vi "Test Find Class from Library.vi"(8 "error in (no error)":errorcluster, 11 "Test Finder Test in":refnum<class "Test Finder Test.lvclass">) -> (0 "error out":errorcluster, 3 "Test Finder Test out":refnum<class "Test Finder Test.lvclass">)   [LabVIEW 2020, in "LUnit Tests.lvlib" / "Test Finder Test.lvclass"]
uses:
  Test Finder Test.lvclass
  C:/Program Files (x86)/National Instruments/LabVIEW 2020/vi.lib/Astemes/LUnit/Test Case.lvclass
  source/Framework/Helper Classes/Test Finder/Test Finder.lvclass
  Test Dummys/Dummy Library/Test Test Case.lvclass
  <vilib>/Astemes/LUnit/Test Case.lvclass/Test Case.ctl
  <vilib>/Astemes/LUnit/LUnit Assertion Result.lvclass/LUnit Assertion Result.ctl
  <vilib>/Astemes/LUnit/LUnit Test Case Result.lvclass/LUnit Test Case Result.ctl
  <vilib>/Astemes/LUnit/LUnit Method Result.lvclass/LUnit Method Result.ctl
  <vilib>/Astemes/LUnit/Palette/Fail.vi
  <vilib>/Astemes/LUnit/Palette/Pass.vi
  <vilib>/Astemes/LUnit/Set Assertion Type.vi
  <vilib>/Astemes/LUnit/Add test result.vi
  <vilib>/Astemes/LUnit/LUnit Write Passed.vi
  <vilib>/Astemes/LUnit/LUnit Write Message.vi
  <vilib>/Astemes/LUnit/LUnit Write Description.vi
  <vilib>/Astemes/LUnit/LUnit Write Assertion Type.vi
  <vilib>/Astemes/LUnit/LUnit Record Assertion Result.vi
  <vilib>/Astemes/LUnit/LUnit Aggregate Assertion Results.vi
  <vilib>/Astemes/LUnit/Assertion Result/LUnit Read Status.vi
  <vilib>/Astemes/LUnit/LUnit Read Message.vi
  <vilib>/Astemes/LUnit/LUnit Read Description.vi
  <vilib>/Astemes/LUnit/Method Result/LUnit Merge Status.vi
  <vilib>/Astemes/LUnit/LUnit Concatenate result strings.vi
  <vilib>/Astemes/LUnit/LUnit Assertion Result.lvclass
  Test Finder Test.lvclass/Test Finder Test.ctl
  <vilib>/Astemes/LUnit/Test Case.lvclass
  C:/Git/astemes-lunit/source/Framework/Test Case/LUnit Test Case.lvclass
  C:/Git/astemes-lunit/tests/Test Dummys/Dummy Library/Test Test Case.lvclass
  C:/Git/astemes-lunit/tests/Test Finder/Test Finder Test.lvclass
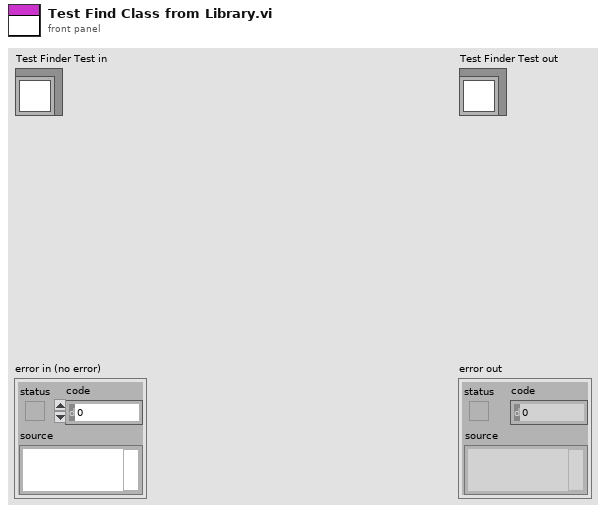
[diagram p1: front panel]
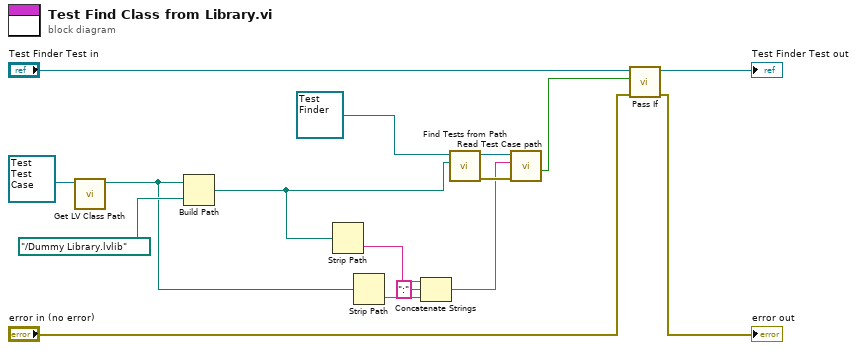
[diagram p0: block diagram]
diagram:
  n1 = call <vilib>:"Get LV Class Path.vi"("object"=refnum<class "Test Test Case.lvclass"> refnum ("Dummy Library.lvlib:Test Test Case.lvclass")) -> ("class path"=w5:path)  [unwired: 9 in, 1 out]
  n2 = Build Path(base path=w5, name or relative path=path "../Dummy Library.lvlib") -> (appended path=w3:path)
  n3 = Strip Path(path=w3) -> (name=w2:string)  [unwired: 1 out]
  n4 = Strip Path(path=w5) -> (name=w9:string)  [unwired: 1 out]
  n5 = Concatenate Strings(w2, ":" ("string"), w9) -> (w4:string)
  n6 = call-dynamic "Find Tests from Path.vi"("Project or Class Path"=w3, "Test Case Finder In"=refnum<class "Test Finder.lvclass"> refnum) -> ("error out"=w11:errorcluster, "Test Case Finder Out"=w12:refnum<class "Test Finder.lvclass">)  [unwired: 8 in]
  n7 = call "Read Test Case path.vi"("error in (no error)"=w11, "Test Case Name"=w4, "Test Case Finder In"=w12) -> ("found?"=w8:bool)  [unwired: 5 in, 3 out]
  n8 = call <vilib>:"Pass If.vi"("error in (no error)"="error in (no error)", "Pass?"=w8, "LUnit Test Case In"="Test Finder Test in") -> ("error out"=→"error out":errorcluster, "LUnit Test Case Out"=→"Test Finder Test out":refnum<class "Test Finder Test.lvclass">)  [unwired: 7 in]
